vi "NATS Start Monitor.vi"(8 "error in":errorcluster, 11 "nats connection in":T1={"connection ID"=refnum, "server INFO"="", "timeout ms"=5000, "verbose?"=FALSE, "server headers?"=FALSE, "client headers?"=FALSE}) -> (0 "error out":errorcluster, 1 "request queue":refnum<queue>, 2 "message queue":refnum<queue>, 3 "async monitor":refnum<vi>)   [LabVIEW 2023, in "NATS Core.lvlib"]
doc: "Reads a message from the NATS server."
uses:
  NATS Core.lvlib
  Controls/nats connection.ctl
  Controls/nats message.ctl
  Controls/msg type.ctl
  NATS Async Monitor.vi
  Controls/request queue.ctl
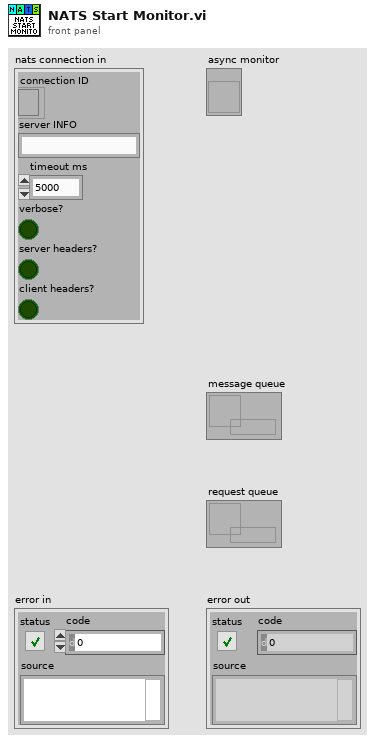
[diagram p1: front panel]
types:
  T1 = typedef "NATS Core.lvlib/nats connection.ctl" = cluster{"connection ID":refnum<k5>, "server INFO":string, "timeout ms":i32, "verbose?":bool, "server headers?":bool, "client headers?":bool}
  T2 = typedef "request queue.ctl" = cluster{"reply subject":string, "request queue":refnum<queue>}
  T3 = typedef "NATS Core.lvlib/nats message.ctl" = cluster{"subject":string, "payload":string, "sub id":string, "reply-to":string, "headers":string, "type":T4, "received":timestamp}
  T4 = typedef "NATS Core.lvlib/msg type.ctl" = enum16{"Undefined", "MSG", "HMSG", "+OK", "PING", "PONG", "-ERR", "INFO"}
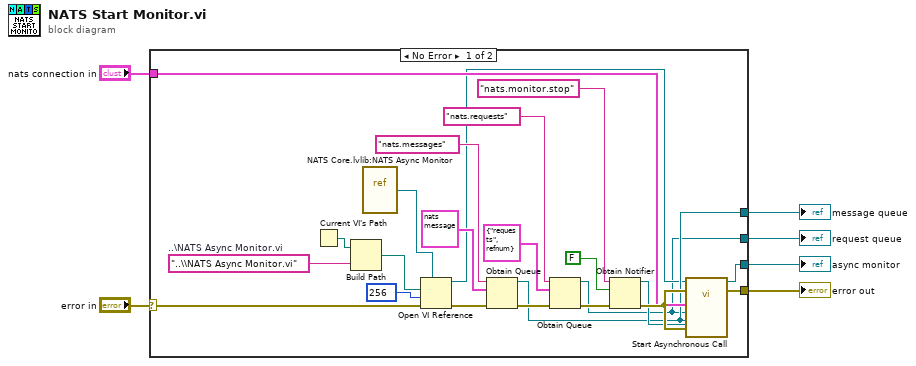
[diagram p0: block diagram]
diagram:
  n1 = case shown="No Error" "error in" {
    selector: "error in" -> [w25 w30]
    tunnel: [w28 w30] -> w5
    tunnel: [w17 _] -> w4
    tunnel: "nats connection in" -> [w16 _]
    tunnel: [w15 _] -> w2
    tunnel: [w7 _] -> w1
    frame No Error {
      w10 = "..\\NATS Async Monitor.vi"  # ..\NATS Async Monitor.vi
      n2 = Current VI's Path() -> (path=w12:path)
      n3 = Build Path(base path=w12, name or relative path=w10) -> (appended path=w9:path)
      n4 = vi-ref "NATS Core.lvlib:NATS Async Monitor.vi"() -> (w14:refnum<vi>)
      n5 = Open VI Reference(type specifier VI Refnum (for type only)=w14, vi path=w9, options=256, error in (no error)=w25) -> (vi reference=w13:refnum<vi>, error out=w24:errorcluster)  [unwired: 2 in]
      n6 = Obtain Queue(name (unnamed)="nats.messages", element data type=T3 {"subject"="", "payload"="", "sub id"="", "reply-to"="", "headers"="", "type"=enum."Undefined", "received"=timestamp(0 s since 1904-01-01)} ("nats message"), error in (no error)=w24) -> (queue out=w15:refnum<queue>, error out=w26:errorcluster)  [unwired: 2 in, 1 out]
      n7 = Obtain Queue(name (unnamed)="nats.requests", element data type=T2 {"reply subject"="requests", "request queue"=refnum}, error in (no error)=w26) -> (queue out=w7:refnum<queue>, error out=w27:errorcluster)  [unwired: 2 in, 1 out]
      n8 = Obtain Notifier(name (unnamed)="nats.monitor.stop", notification data type=FALSE, error in (no error)=w27) -> (notifier out=w18:refnum<notifier>, error out=w29:errorcluster)  [unwired: 1 in, 1 out]
      n9 = call-by-ref "Start Asynchronous Call"(reference=w13, error in=w29, "stop"=w18, "error in"=w29, "message queue"=w15, "request queue"=w7, "nats connection in"=w16) -> (reference out=w17:refnum<vi>, error out=w28:errorcluster)  [unwired: 6 in, 1 out]
    }
    frame Error {
    }
  }
  "error out" <- w5
  "async monitor" <- w4
  "message queue" <- w2
  "request queue" <- w1
